vi "MaxiGauge EPICSorg.vi"() -> ()   [LabVIEW 2015]
uses:
  <vilib>/Platform/TimedLoop/XDataNode/timing_clust.ctl
  <vilib>/Platform/TimedLoop/XDataNode/nitl_modes.ctl
  <vilib>/Platform/TimedLoop/XDataNode/wakeup.ctl
  <userlib>/caLab/Private/Get_PV-1D.vi
  <userlib>/caLab/Private/Put_DBL-1D_PV-1D.vi
  <vilib>/platform/TimedLoop/XDataNode/XDataNode.xnode
  <vilib>/Platform/TimedLoop/XDataNode/XDNodeRunTimeDep.lvlib
panel:
  out "Boolean array":bool[](array[boolean])
  out "Maxigauge COMPORT":string
  out "concatenated string":string
  out "APX:SEN6_STS":bool
  out "APX:SEN5_STS":bool
  out "APX:SEN4_STS":bool
  out "APX:SEN3_STS":bool
  out "APX:SEN2_STS":bool
  out "APX:SEN1_STS":bool
  out "APX:SEN6_VAL":dbl
  out "APX:SEN5_VAL":dbl
  out "APX:SEN4_VAL":dbl format="%#_3g"
  out "APX:SEN3_VAL":dbl format="%#_3g"
  out "APX:SEN2_VAL":dbl format="%#_3g"
  out "APX:SEN1_VAL":dbl
  in  "APX:SEN6_OFF":bool
  in  "APX:SEN6_ON":bool
  in  "APX:SEN5_OFF":bool
  in  "APX:SEN5_ON":bool
  in  "APX:SEN4_OFF":bool
  in  "APX:SEN4_ON":bool
  in  "APX:SEN3_OFF":bool
  in  "APX:SEN3_ON":bool
  in  "APX:SEN2_OFF":bool
  in  "APX:SEN2_ON":bool
  in  "APX:SEN1_OFF":bool
  in  "APX:SEN1_ON":bool
  out "APX:SP_SES100":bool
  out "MaxiGauge":dbl[](array[numeric])
  out "P torr":dbl[](array[numeric])
  in  "STOP":bool
  # "Ch 1\nGMP\nCh 6\nGMP\nCh 2\nGCC\nCh 4\nGHC\nCh 5\nGHC\n\nGMP"
  # "Send measured values to EPICS [COM8]"
  # "K"
  # "EPICS PV name"
  # "N"
  # "APX:HPC100"
  # "APX:HPC100"
  # "APX:HPC01"
  # "APX:HPC"
  # "APX:HPC"
  # "N"
  # "APX:AP1"
  # "APX:PREP"
  # "APX:AP2"
  # "APX:Tsample"
  # "APX:AP1"
  # "APX:Tpiezo"
  # "APX:Thpc"
  # "APX:AP2"
  # "APX:PREP"
  # "APX:HPC01"
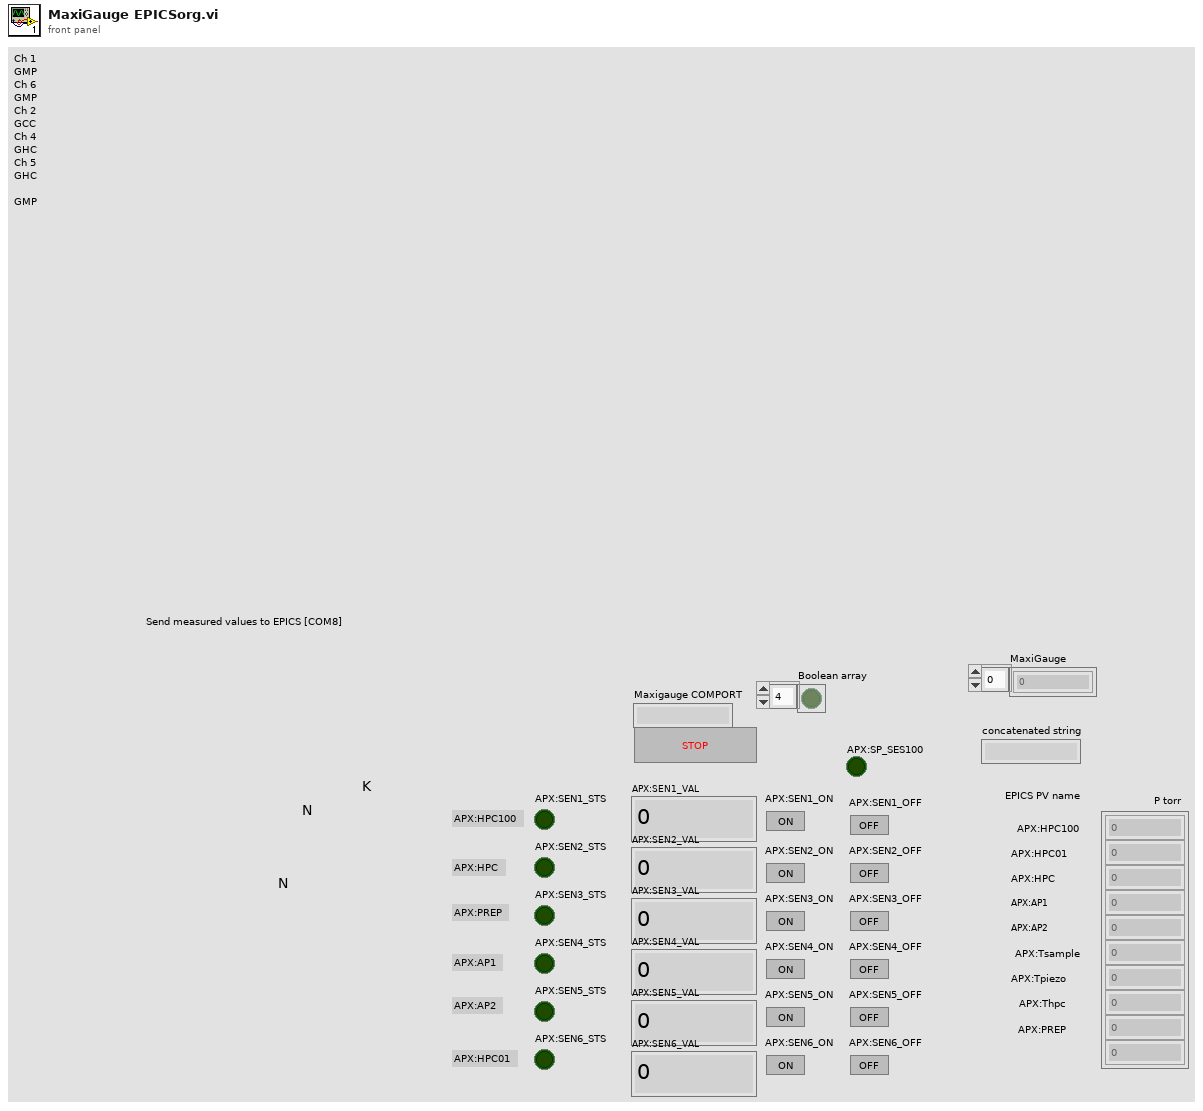
[diagram p1: front panel]
types:
  T1 = typedef "XDNodeRunTimeDep.lvlib/timing_clust.ctl" = cluster{"Expected End [f-1]":u64, "Actual End [f-1]":u64, "Finished Late? [f-1]":bool, "Expected End [i-1]":u64, "Actual End [i-1]":u64, "Finished Late? [i-1]":bool, "Expected Start [i]":u64, "Actual Start [i]":u64, "Expected Start [f]":u64, "Actual Start [f]":u64, "Source Name":string, "Structure Name":string, "Period":i64, "Deadline":i64, "Offset":i64, "Start":i64, "Priority":i32, "Timeout":i32, "Mode":T2, "Wakeup Reason":T3, "Error":errorcluster, "Source Type":string, "Secondary Source Type":string, "Global End Time":u64, "Global Start Time":u64, "Frame Duration":u64, "Iteration Duration":u64, "Assigned CPU":i32, "I/O Scan Engine Mode":u32}
  T2 = typedef "XDNodeRunTimeDep.lvlib/nitl_modes.ctl" = enum32{"No Change", "Process missed periods, maintain original phase", "Discard missed periods, maintain original phase", "Process missed periods, ignore original phase", "Discard missed periods, ignore original phase"}
  T3 = typedef "XDNodeRunTimeDep.lvlib/wakeup.ctl" = enum32{"Normal", "Aborted", "Asynchronous wakeup", "Timing source error", "Timed loop error", "Timeout"}
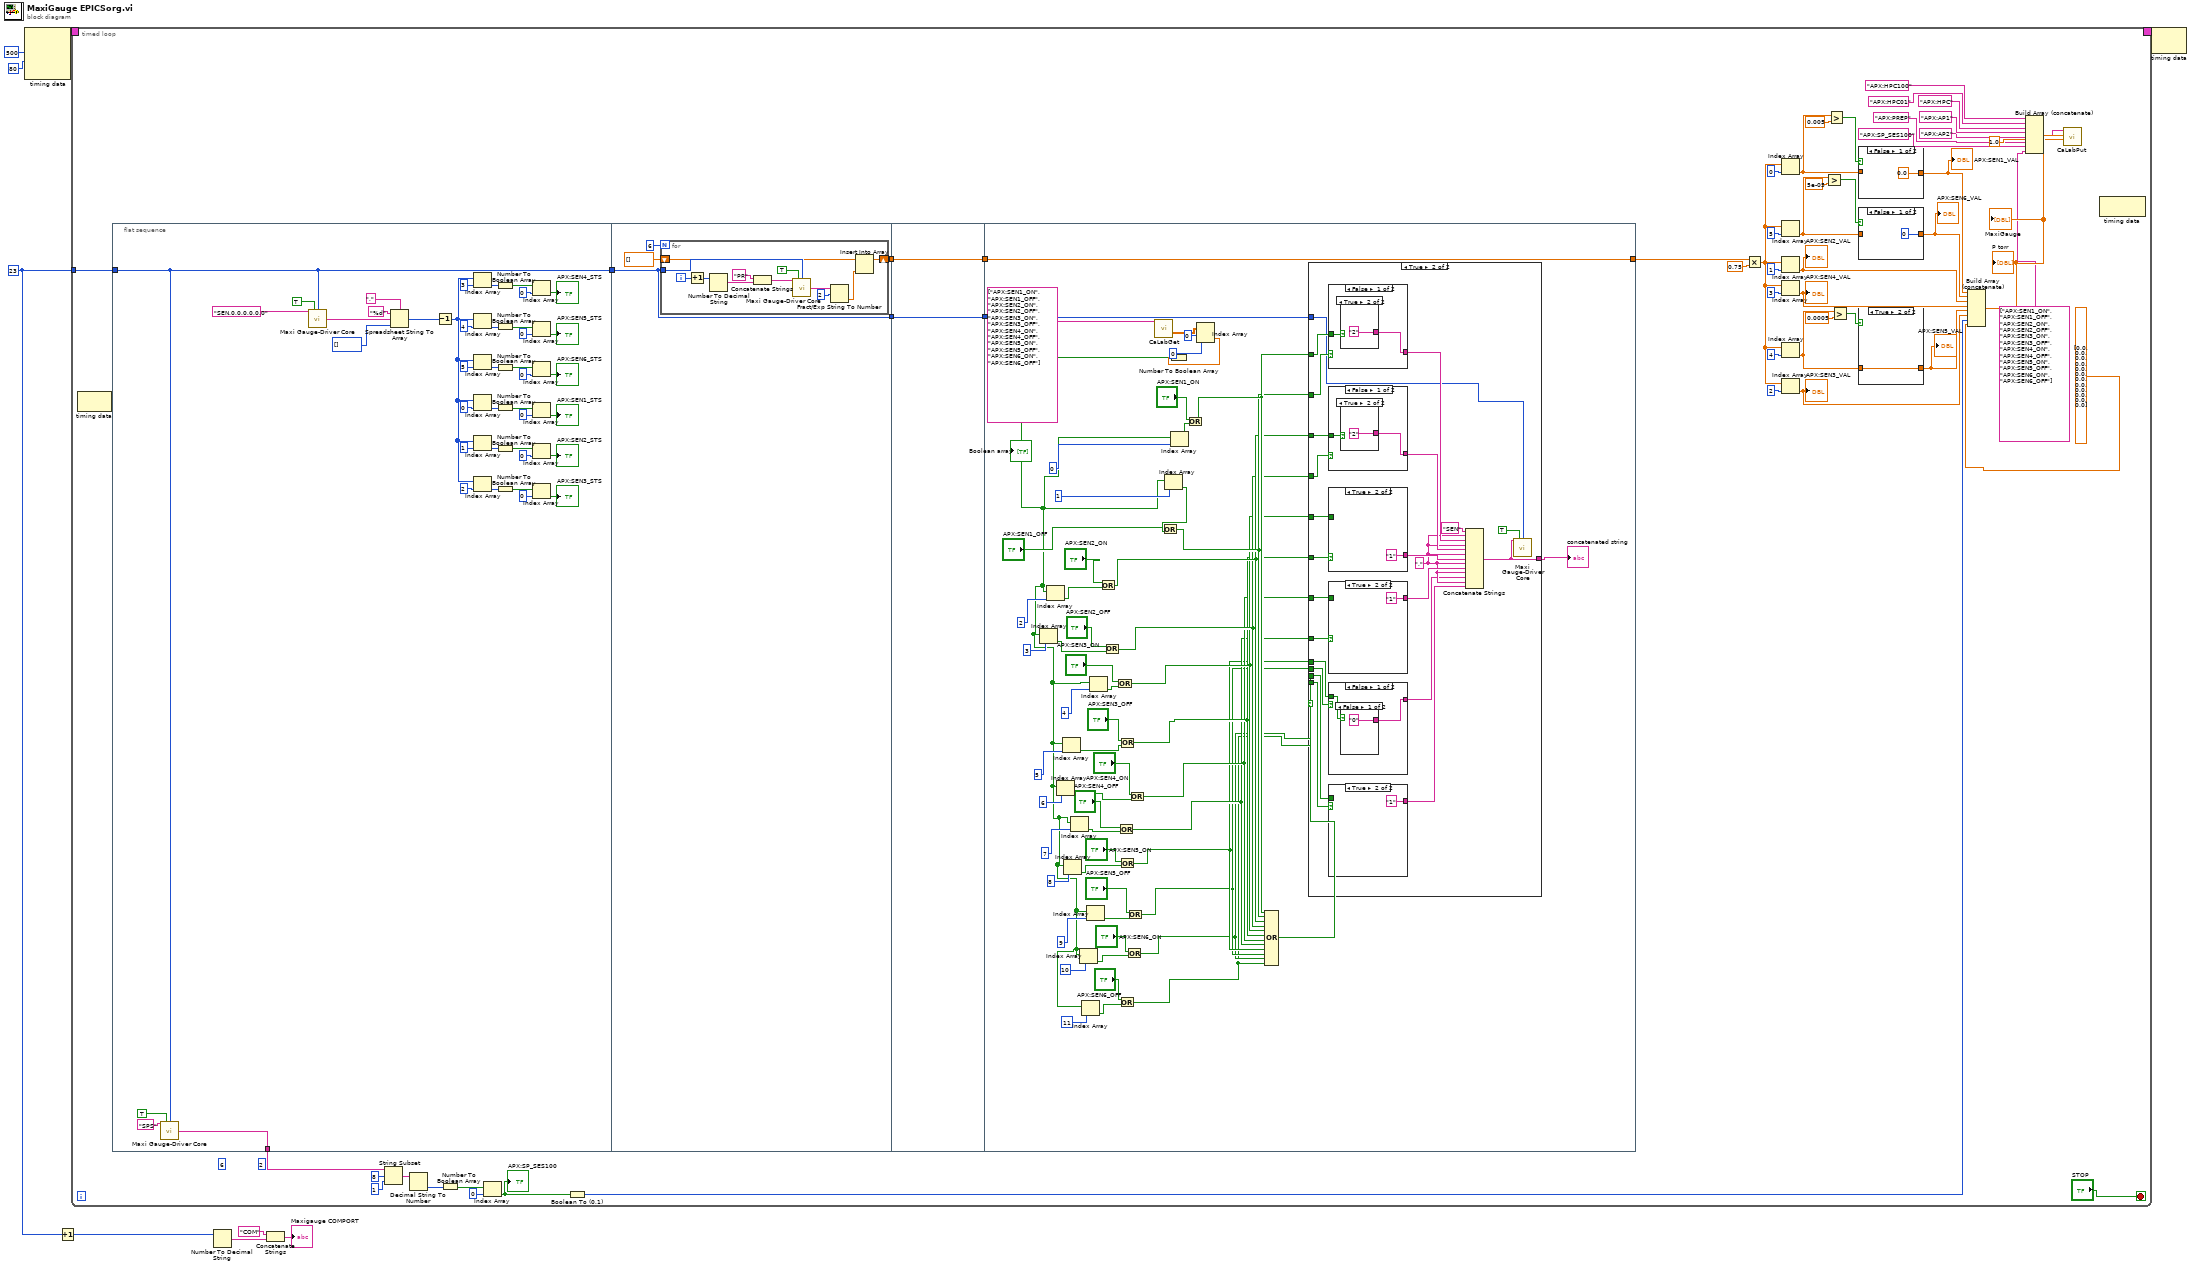
[diagram p0: block diagram]
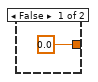
[diagram p2: hidden frame]
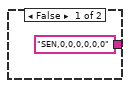
[diagram p3: hidden frame]
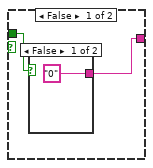
[diagram p4: hidden frame]
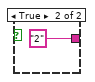
[diagram p5: hidden frame]
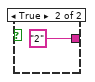
[diagram p6: hidden frame]
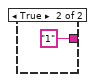
[diagram p7: hidden frame]
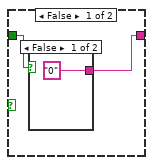
[diagram p8: hidden frame]
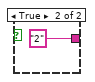
[diagram p9: hidden frame]
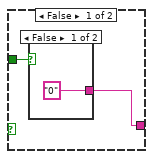
[diagram p10: hidden frame]
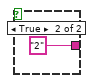
[diagram p11: hidden frame]
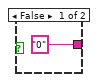
[diagram p12: hidden frame]
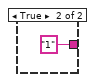
[diagram p13: hidden frame]
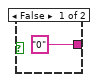
[diagram p14: hidden frame]
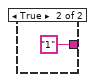
[diagram p15: hidden frame]
diagram:
  w5 = 23 ("Port")
  n1 = node-c288(i64 500 ("Period"), 80 ("Priority")) -> (w9:T1)  [unwired: 2 in]
  n2 = Increment(x=w5) -> (x+1=w4:i32)
  n3 = timed-loop {
    tunnel: w5 -> [w39]
    timing: w9 -> [_]
    timing-out: [_] -> w8
    stop <- "STOP" stop-if-true
    (unwired) 6
    (unwired) 2 ("index")
    n4 = node-c288() -> ()  [unwired: 1 in, 1 out]
    n5 = flat-sequence {
      tunnel: w39 -> [w100]
      tunnel: [w100] -> w38
      tunnel: [w103] -> w35
      tunnel: w38 -> [w106]
      tunnel: [w107] -> w15
      tunnel: [w106] -> w13
      tunnel: w15 -> [w123]
      tunnel: [w123] -> w14
      tunnel: w13 -> [w122]
      tunnel: [w122] -> w12
      tunnel: [w181] -> w51
      tunnel: w14 -> [w181]
      tunnel: w12 -> [w178]
      frame #0 {
        n6 = call "Maxi Gauge-Driver Core.vi"("Command"="SPS", "Write/Read"=TRUE, "Port"=w100) -> ("String Out"=w103:string)  [unwired: 3 in, 9 out]
        n7 = call "Maxi Gauge-Driver Core.vi"("Command"="SEN,0,0,0,0,0,0", "Write/Read"=TRUE, "Port"=w100) -> ("String Out"=w98:string)  [unwired: 3 in, 9 out]
        n8 = Spreadsheet String To Array(delimiter (Tab)=",", format string="%d", spreadsheet string=w98, array type (2D Dbl)=i16[] []) -> (array=w94:i16[])
        n9 = Decrement(x=w94) -> (x-1=w69:i16[])
        n10 = Index Array(array=w69, index=3) -> (element=w80:i16)
        n11 = Index Array(array=w69, index=4) -> (element=w76:i16)
        n12 = Index Array(array=w69, index=5) -> (element=w72:i16)
        n13 = Index Array(array=w69, index=0) -> (element=w93:i16)
        n14 = Index Array(array=w69, index=1) -> (element=w88:i16)
        n15 = Index Array(array=w69, index=2) -> (element=w84:i16)
        n16 = Number To Boolean Array(number=w80) -> (Boolean array=w79:bool[])
        n17 = Number To Boolean Array(number=w76) -> (Boolean array=w75:bool[])
        n18 = Number To Boolean Array(number=w72) -> (Boolean array=w71:bool[])
        n19 = Number To Boolean Array(number=w93) -> (Boolean array=w92:bool[])
        n20 = Number To Boolean Array(number=w88) -> (Boolean array=w87:bool[])
        n21 = Number To Boolean Array(number=w84) -> (Boolean array=w83:bool[])
        n22 = Index Array(array=w79, index=0) -> (element=→"APX:SEN4_STS":bool)
        n23 = Index Array(array=w75, index=0) -> (element=→"APX:SEN5_STS":bool)
        n24 = Index Array(array=w71, index=0) -> (element=→"APX:SEN6_STS":bool)
        n25 = Index Array(array=w92, index=0) -> (element=→"APX:SEN1_STS":bool)
        n26 = Index Array(array=w87, index=0) -> (element=→"APX:SEN2_STS":bool)
        n27 = Index Array(array=w83, index=0) -> (element=→"APX:SEN3_STS":bool)
      }
      frame #1 {
        n28 = for {
          N: 6 -> [_]
          tunnel: w106 -> [w113]
          shift-right: [w110] -> w107
          shift-left: dbl[] [] -> [w111]
          i -> [w115]
          n29 = Increment(x=w115) -> (x+1=w118:i32)
          n30 = Number To Decimal String(number=w118) -> (decimal integer string=w121:string)  [unwired: 1 out]
          n31 = Concatenate Strings("PR", w121) -> (w119:string)
          n32 = call "Maxi Gauge-Driver Core.vi"("Command"=w119, "Write/Read"=TRUE, "Port"=w113) -> ("String Out"=w117:string)  [unwired: 3 in, 9 out]
          n33 = Fract/Exp String To Number(string=w117, offset=2 ("offset (0)")) -> (number=w112:dbl)  [unwired: 3 out]
          n34 = Insert Into Array(array=w111, new element=w112) -> (w110:dbl[])  [unwired: 1 in]
        }
      }
      frame #2 {
      }
      frame #3 {
        n35 = call-poly "CaLabGet.vi"("PV Names"=string[] ["APX:SEN1_ON", "APX:SEN1_OFF", "APX:SEN2_ON", "APX:SEN2_OFF", "APX:SEN3_ON", "APX:SEN3_OFF", "APX:SEN4_ON", "APX:SEN4_OFF", "APX:SEN5_ON", "APX:SEN5_OFF", "APX:SEN6_ON", "APX:SEN6_OFF"]) -> ("Value Array (number)"=w174:dbl[][])  [unwired: 8 in, 6 out]
        n36 = Index Array(array=w174, index (row)=0, index (col)=0 ("disabled index (col)")) -> (element=w177:dbl)
        n37 = Number To Boolean Array(number=w177) -> (Boolean array=w148:bool[])
        "Boolean array" <- w148
        n38 = Index Array(array=w148, index=3) -> (element=w154:bool)
        n39 = Index Array(array=w148, index=2) -> (element=w155:bool)
        n40 = Index Array(array=w148, index=6) -> (element=w141:bool)
        n41 = Index Array(array=w148, index=5) -> (element=w144:bool)
        n42 = Index Array(array=w148, index=8) -> (element=w135:bool)
        n43 = Index Array(array=w148, index=7) -> (element=w138:bool)
        n44 = Index Array(array=w148, index=10) -> (element=w133:bool)
        n45 = Index Array(array=w148, index=11) -> (element=w132:bool)
        n46 = Index Array(array=w148, index=9) -> (element=w134:bool)
        n47 = Index Array(array=w148, index=4) -> (element=w147:bool)
        n48 = Or(x="APX:SEN2_ON", y=w155) -> (x .or. y?=w152:bool)
        n49 = Or(x="APX:SEN2_OFF", y=w154) -> (x .or. y?=w151:bool)
        n50 = Or(x="APX:SEN3_ON", y=w147) -> (x .or. y?=w145:bool)
        n51 = Or(x="APX:SEN4_OFF", y=w138) -> (x .or. y?=w136:bool)
        n52 = Or(x="APX:SEN6_OFF", y=w132) -> (x .or. y?=w124:bool)
        n53 = Or(x="APX:SEN3_OFF", y=w144) -> (x .or. y?=w142:bool)
        n54 = Or(x="APX:SEN5_ON", y=w135) -> (x .or. y?=w130:bool)
        n55 = Or(x="APX:SEN6_ON", y=w133) -> (x .or. y?=w126:bool)
        n56 = Or(x="APX:SEN5_OFF", y=w134) -> (x .or. y?=w128:bool)
        n57 = Or(x="APX:SEN4_ON", y=w141) -> (x .or. y?=w139:bool)
        n58 = Index Array(array=w148, index=1) -> (element=w167:bool)
        n59 = Or(x="APX:SEN1_OFF", y=w167) -> (x .or. y?=w165:bool)
        n60 = Index Array(array=w148, index=0) -> (element=w170:bool)
        n61 = Or(x="APX:SEN1_ON", y=w170) -> (x .or. y?=w168:bool)
        n62 = Compound Arithmetic op=OR(w168, w165, w152, w151, w145, w142, w139, w136, w130, w128, w126, w124) -> (w179:bool)
        n63 = case shown="True" w179 {
          tunnel: w165 -> [_ w204]
          tunnel: w168 -> [_ w203]
          tunnel: w152 -> [_ w202]
          tunnel: w151 -> [_ w201]
          tunnel: w145 -> [_ w200]
          tunnel: w142 -> [_ w199]
          tunnel: w136 -> [_ w198]
          tunnel: w139 -> [_ w197]
          tunnel: w130 -> [_ w196]
          tunnel: w128 -> [_ w195]
          tunnel: w126 -> [_ w194]
          tunnel: w124 -> [_ w193]
          tunnel: ["SEN,0,0,0,0,0,0" w185] -> w180
          tunnel: w178 -> [_ w183]
          frame False {
          }
          frame True {
            w188 = "," ("string")
            n64 = case shown="False" w204 {
              tunnel: w203 -> [w232 _]
              tunnel: [w231 "1"] -> w192
              frame False {
                n65 = case shown="True" w232 {
                  tunnel: ["0" "2"] -> w231
                  frame False {
                  }
                  frame True {
                  }
                }
              }
              frame True {
              }
            }
            n66 = case shown="False" w201 {
              tunnel: w202 -> [w227 _]
              tunnel: [w226 "1"] -> w191
              frame False {
                n67 = case shown="True" w227 {
                  tunnel: ["0" "2"] -> w226
                  frame False {
                  }
                  frame True {
                  }
                }
              }
              frame True {
              }
            }
            n68 = case shown="True" w199 {
              tunnel: w200 -> [w222 _]
              tunnel: [w221 "1"] -> w190
              frame False {
                n69 = case shown="False" w222 {
                  tunnel: ["0" "2"] -> w221
                  frame False {
                  }
                  frame True {
                  }
                }
              }
              frame True {
              }
            }
            n70 = case shown="True" w198 {
              tunnel: w197 -> [w217 _]
              tunnel: [w216 "1"] -> w189
              frame False {
                n71 = case shown="False" w217 {
                  tunnel: ["0" "2"] -> w216
                  frame False {
                  }
                  frame True {
                  }
                }
              }
              frame True {
              }
            }
            n72 = case shown="False" w195 {
              tunnel: w196 -> [w212 _]
              tunnel: [w211 "1"] -> w187
              frame False {
                n73 = case shown="False" w212 {
                  tunnel: ["0" "2"] -> w211
                  frame False {
                  }
                  frame True {
                  }
                }
              }
              frame True {
              }
            }
            n74 = case shown="True" w193 {
              tunnel: w194 -> [w207 _]
              tunnel: [w206 "1"] -> w186
              frame False {
                n75 = case shown="False" w207 {
                  tunnel: ["0" "2"] -> w206
                  frame False {
                  }
                  frame True {
                  }
                }
              }
              frame True {
              }
            }
            n76 = Concatenate Strings("SEN", w188, w192, w188, w191, w188, w190, w188, w189, w188, w187, w188, w186) -> (w185:string)
            n77 = call "Maxi Gauge-Driver Core.vi"("Command"=w185, "Write/Read"=TRUE, "Port"=w183) -> ()  [unwired: 3 in, 10 out]
          }
        }
        "concatenated string" <- w180
      }
    }
    n78 = String Subset(string=w35, offset (0)=8, length (rest)=1 ("length (rest)")) -> (substring=w31:string)
    n79 = Decimal String To Number(string=w31) -> (number=w32:i32)  [unwired: 2 in, 1 out]
    n80 = Number To Boolean Array(number=w32) -> (Boolean array=w34:bool[])
    n81 = Index Array(array=w34, index=0) -> (element=w30:bool)
    "APX:SP_SES100" <- w30
    n82 = Boolean To (0,1)(Boolean=w30) -> (0, 1=w21:i16)
    n83 = Multiply(x=w51, y=0.75) -> (x*y=w41:dbl[])
    n84 = Index Array(array=w41, index=0) -> (element=w29:dbl)
    n85 = Index Array(array=w41, index=5) -> (element=w26:dbl)
    n86 = Index Array(array=w41, index=1) -> (element=w28:dbl)
    "APX:SEN2_VAL" <- w28
    n87 = Index Array(array=w41, index=3) -> (element=w27:dbl)
    "APX:SEN4_VAL" <- w27
    n88 = Index Array(array=w41, index=4) -> (element=w19:dbl)
    n89 = Index Array(array=w41, index=2) -> (element=w23:dbl)
    "APX:SEN3_VAL" <- w23
    n90 = Greater?(x=w26, y=5e-05) -> (0:w55:bool)
    n91 = Greater?(x=w29, y=0.005) -> (0:w52:bool)
    n92 = Greater?(x=w19, y=0.0005) -> (0:w20:bool)
    n93 = case shown="False" w52 {
      tunnel: [0.0 w237] -> w16
      tunnel: w29 -> [_ w237]
      frame False {
      }
      frame True {
      }
    }
    "APX:SEN1_VAL" <- w16
    n94 = case shown="False" w55 {
      tunnel: [0 w239] -> w17
      tunnel: w26 -> [_ w239]
      frame False {
      }
      frame True {
      }
    }
    "APX:SEN6_VAL" <- w17
    n95 = case shown="True" w20 {
      tunnel: [0.0 w63] -> w18
      tunnel: w19 -> [_ w63]
      frame False {
      }
      frame True {
      }
    }
    "APX:SEN5_VAL" <- w18
    n96 = Build Array (concatenate)(w16, w17, w28, w27, w18, w23, w21, dbl[] [0.0, 0.0, 0.0, 0.0, 0.0, 0.0, 0.0, 0.0, 0.0, 0.0, 0.0, 0.0]) -> (w49:dbl[])
    "P torr" <- w49
    "MaxiGauge" <- w49
    n97 = Build Array (concatenate)("APX:HPC100", "APX:HPC01", "APX:HPC", "APX:AP1", "APX:AP2", "APX:PREP", "APX:SP_SES100" ("element"), string[] ["APX:SEN1_ON", "APX:SEN1_OFF", "APX:SEN2_ON", "APX:SEN2_OFF", "APX:SEN3_ON", "APX:SEN3_OFF", "APX:SEN4_ON", "APX:SEN4_OFF", "APX:SEN5_ON", "APX:SEN5_OFF", "APX:SEN6_ON", "APX:SEN6_OFF"]) -> (w48:string[])
    n98 = call-poly <userlib>:"CaLabPut.vi"("Timeout (3)"=1.0, "Values"=w49, "PV Names"=w48) -> ()  [unwired: 5 in, 4 out]
    n99 = node-c288() -> ()  [unwired: 1 in, 1 out]
  }
  n100 = Number To Decimal String(number=w4) -> (decimal integer string=w3:string)  [unwired: 1 in]
  n101 = Concatenate Strings("COM" ("string"), w3) -> (→"Maxigauge COMPORT":string)
  n102 = node-c288(w8) -> ()  [unwired: 1 out]
